vi "Evaluate.vi"(8 "error in (no error)":errorcluster, 10 "Data":refnum<class "Data.lvclass">[](array[class]), 11 "Data Tracker Msg in":refnum<class "Data Tracker Msg.lvclass">) -> (0 "error out":errorcluster, 3 "Tracker Data":refnum<class "Tracker Data.lvclass">)   [LabVIEW 2020, in "Data Tracker.lvlib" / "Data Tracker Msg.lvclass"]
doc: "Evaluate the tracked Data and return Tracker Data.\n\nThe parent implementation does nothing."
uses:
  Data Tracker Msg.lvclass
  PPL/HDH.Data.Generic.lvlibp/Data.lvclass
  Data Tracker/Data/Tracker Data.lvclass
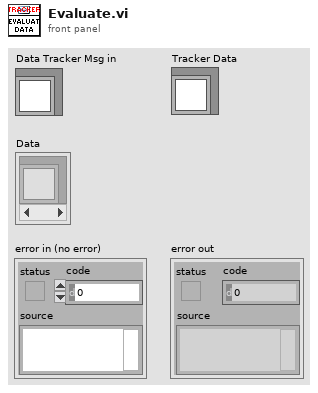
[diagram p1: front panel]
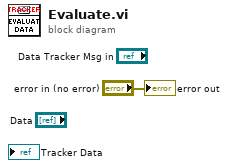
[diagram p0: block diagram]
diagram:
  "error out" <- "error in (no error)"
